vi "Read Get Device Parameter Status.vi"(11 "Get Device Parameter Status Msg in":refnum<class "Get Device Parameter Status Msg.lvclass">) -> (0 "Status":T1, 1 "Parameter Name":string, 2 "IED Name":string, 3 "Get Device Parameter Status Msg out":refnum<class "Get Device Parameter Status Msg.lvclass">, 4 "Parameter/Error":string)   [LabVIEW 2015, in "SCADA Core.lvlib" / "Get Device Parameter Status Msg.lvclass"]
uses:
  Get Device Parameter Status Msg.lvclass
  Get Device Parameter Status.ctl
  Get Device Parameter Status Msg.lvclass/Get Device Parameter Status Msg.ctl
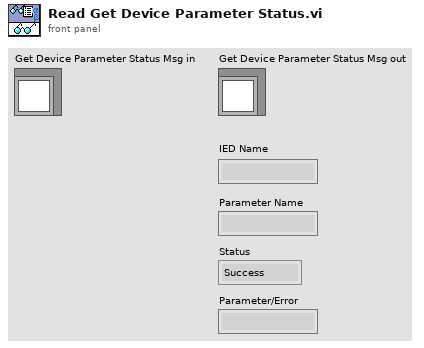
[diagram p1: front panel]
types:
  T1 = typedef "SCADA Core.lvlib/Get Device Parameter Status Msg.lvclass/Get Device Parameter Status.ctl" = enum16{"Success", "Failure"}
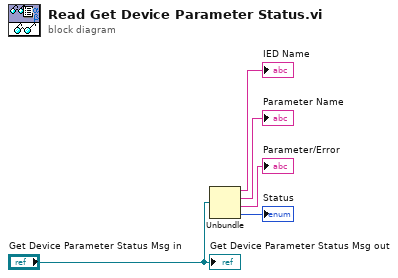
[diagram p0: block diagram]
diagram:
  n1 = Unbundle("Get Device Parameter Status Msg in") -> (→"IED Name":string, →"Parameter Name":string, →"Parameter/Error":string, →"Status":T1)
  "Get Device Parameter Status Msg out" <- "Get Device Parameter Status Msg in"
